vi "TransducerTypeInformation.vi"(8 "error in (no error)":errorcluster, 11 "Connection Data In":T2) -> (0 "error out":errorcluster, 2 "Cluster Calibration":T1, 3 "Connection Data Out":T2)   [LabVIEW 2014, in "MSX-E3711_dll.lvlib"]
doc: "Recorre la memoria del Data base buscando la información de los transductores que esta misma aloja, adquiere la información de cada uno y los envía al Clúster de Calibración."
uses:
  MSX-E3711_dll.lvlib
  Typedef/Connection Data.ctl
  E:/Repositorio Magnis/INF002/v0/Modules/HAL/Drivers/Sync/ADDI-DATA MSX-E3711/API/MSXE371x.dll
  MSXE371x.dll
  E:/Repositorio Magnis/INF002/v0/Modules/HAL/Drivers/Sync/ADDI-DATA MSX-E3711/API/MXCommon.dll
  MXCommon.dll
  Typedef/Calibration Data.ctl
panel:
  # "Information"
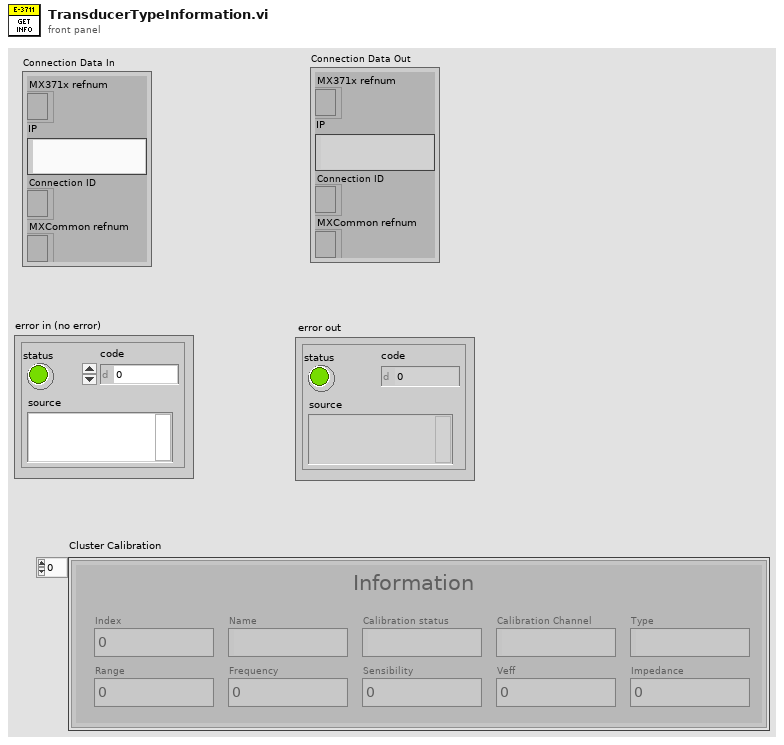
[diagram p1: front panel]
types:
  T1 = typedef "MSX-E3711_dll.lvlib/Calibration Data.ctl" = cluster{"Calibration status":string, "Name":string, "Index":u64, "Range":dbl, "Sensibility":dbl, "Veff":dbl, "Frequency":u64, "Impedance":u64, "Type":string, "Calibration Channel":string}[]
  T2 = typedef "MSX-E3711_dll.lvlib/Connection Data.ctl" = cluster{"MX371x refnum":refnum<k24>, "IP":string, "Connection ID ":refnum<k5>, "MXCommon refnum":refnum<k24>}
  T3 = cluster{"Calibration status":string, "Name":string, "Index":u64, "Range":dbl, "Sensibility":dbl, "Veff":dbl, "Frequency":u64, "Impedance":u64, "Type":string, "Calibration Channel":string}
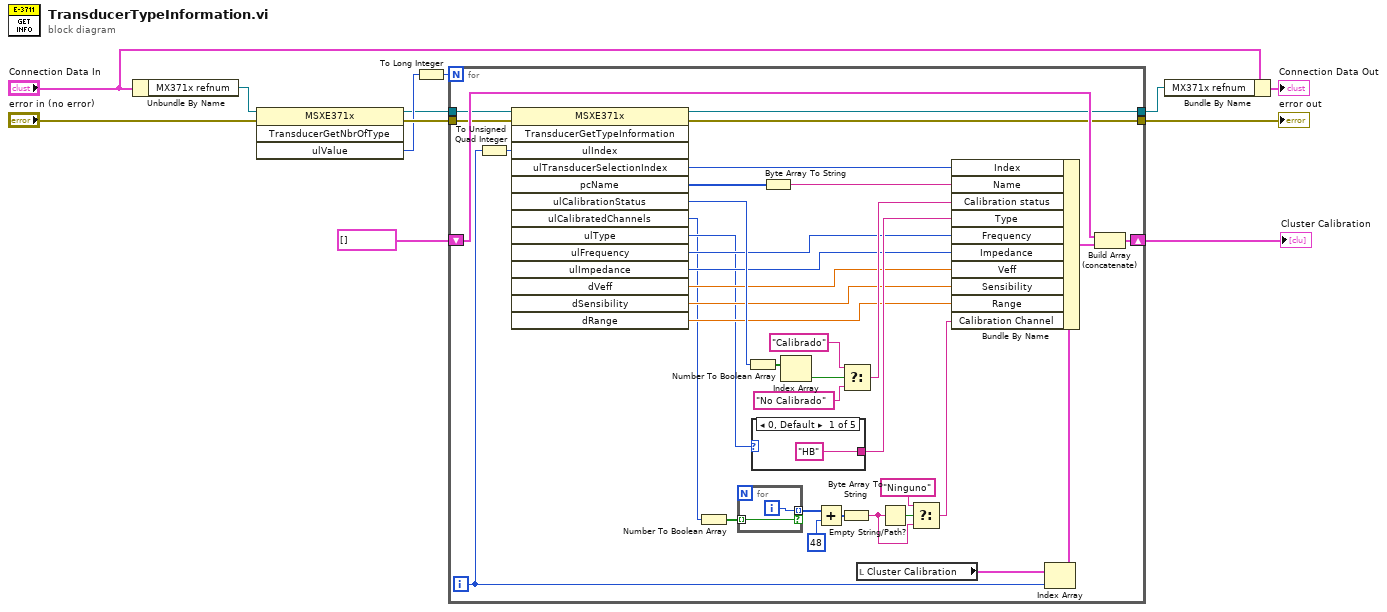
[diagram p0: block diagram]
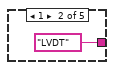
[diagram p2: hidden frame]
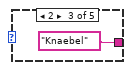
[diagram p3: hidden frame]
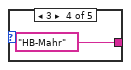
[diagram p4: hidden frame]
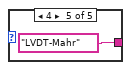
[diagram p5: hidden frame]
diagram:
  n1 = Unbundle By Name("Connection Data In") -> ("MX371x refnum"=w1:refnum<k24>)
  n2 = invoke class="MSXE371x" method="TransducerGetNbrOfType"(reference=w1, error in="error in (no error)") -> (reference out=w2:refnum<k24>, error out=w4:errorcluster, "ulValue"=w3:u64)  [unwired: 2 in, 1 out]
  n3 = To Long Integer(number=w3) -> (32bit integer=w9:i32)
  n4 = for {
    N: w9 -> [_]
    tunnel: w2 -> [w22]
    tunnel: w4 -> [w34]
    tunnel: [w23] -> w8
    tunnel: [w35] -> w10
    shift-right: [w43] -> w7
    shift-left: T1 [] ("Cluster Calibration 2") -> [w42]
    i -> [w45]
    n5 = To Unsigned Quad Integer(1:w45) -> (0:w33:u64)
    n6 = invoke class="MSXE371x" method="TransducerGetTypeInformation"(reference=w22, error in=w34, "ulIndex"=w33) -> (reference out=w23:refnum<k24>, error out=w35:errorcluster, "ulTransducerSelectionIndex"=w32:u64, "pcName"=w31:u8[], "ulCalibrationStatus"=w30:u64, "ulCalibratedChannels"=w17:u64, "ulType"=w24:u64, "ulFrequency"=w25:u64, "ulImpedance"=w26:u64, "dVeff"=w27:dbl, "dSensibility"=w28:dbl, "dRange"=w29:dbl)  [unwired: 11 in, 2 out]
    n7 = Number To Boolean Array(number=w17) -> (Boolean array=w18:bool[])
    n8 = for {
      tunnel: [w50] -> w19 mode=indexing if=w49
      tunnel: w18 -> [w49] mode=indexing
      i -> [w50]
    }
    n9 = Number To Boolean Array(number=w30) -> (Boolean array=w38:bool[])
    n10 = case shown="0, Default" w24 {
      tunnel: ["HB" "LVDT" "Knaebel" "HB-Mahr" "LVDT-Mahr"] -> w36
      frame 0, Default {
      }
      frame 1 {
      }
      frame 2 {
      }
      frame 3 {
      }
      frame 4 {
      }
    }
    n11 = Byte Array To String(unsigned byte array=w31) -> (string=w48:string)
    n12 = Index Array(array=w38) -> (element=w37:bool)  [unwired: 1 in]
    n13 = Add(x=w19, y=48 ("Numeric")) -> (x+y=w21:i32[])
    n14 = Byte Array To String(unsigned byte array=w21) -> (string=w15:string)
    n15 = Select(t="Calibrado", s=w37, f="No Calibrado") -> (s? t:f=w41:string)
    n16 = local read "Cluster Calibration"() -> (w47:T1)
    n17 = Empty String/Path?(string/path=w15) -> (empty?=w16:bool)
    n18 = Select(t="Ninguno", s=w16, f=w15) -> (s? t:f=w14:string)
    n19 = Index Array(array=w47, index=w45) -> (element=w46:T3)
    n20 = Bundle By Name(cluster=w46, "Index"=w32, "Name"=w48, "Calibration status"=w41, "Type"=w36, "Frequency"=w25, "Impedance"=w26, "Veff"=w27, "Sensibility"=w28, "Range"=w29, "Calibration Channel"=w14) -> (w44:T3)
    n21 = Build Array (concatenate)(w42, w44) -> (w43:T1)
  }
  "error out" <- w10
  "Cluster Calibration" <- w7
  n22 = Bundle By Name(cluster="Connection Data In", "MX371x refnum"=w8) -> (→"Connection Data Out":T2)
